vi "InitCAN.vi"(8 "error in (no error)":errorcluster, 10 "Channel Num":T1, 11 "Class-Interface in":refnum<class "Class-Interface.lvclass">) -> (0 "error out":errorcluster, 3 "Class-Interface out":refnum<class "Class-Interface.lvclass">)   [LabVIEW 2019, in "CAN-Interface.lvlib" / "Class-Interface.lvclass"]
uses:
  Class-Interface.lvclass
  TypeDef/Def-ChannelNum.ctl
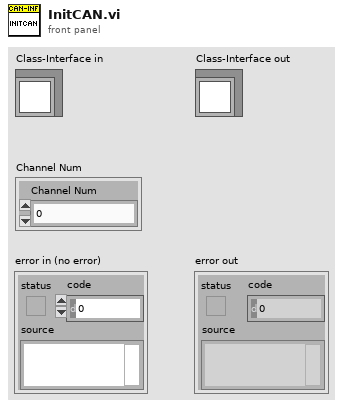
[diagram p1: front panel]
types:
  T1 = typedef "CAN-Interface.lvlib/Class-Interface.lvclass/Def-ChannelNum.ctl" = cluster{"Channel Num":u32}
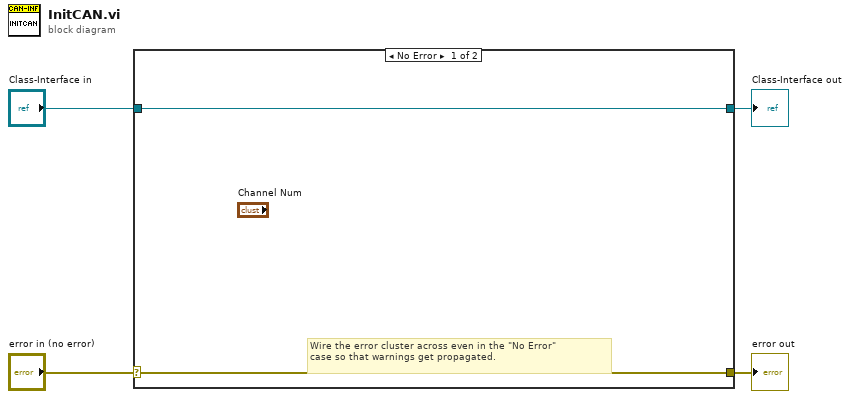
[diagram p0: block diagram]
diagram:
  n1 = case shown="No Error" "error in (no error)" {
    selector: "error in (no error)" -> [w5 w8]
    tunnel: [w5 w8] -> w3
    tunnel: [w6 w7] -> w1
    tunnel: "Class-Interface in" -> [w6 w7]
    frame No Error {
      # "Wire the error cluster across even in the \"No Error\"\ncase so that warnings get propagated."
    }
    frame Error {
    }
  }
  "error out" <- w3
  "Class-Interface out" <- w1
